vi "TrueRMS.vi"(9 "millisecond multiple":u32, 10 "task/channels in":refnum<k21>) -> (4 "Average":dbl[](graph), 6 "spreadsheet string":string)   [LabVIEW 2021]
uses:
  <vilib>/DAQmx/read.llb/DAQmx Read (Analog 1D Wfm NChan NSamp).vi
  <vilib>/DAQmx/miscellaneous.llb/DAQmx Fill In Error Info.vi
  <vilib>/measure/madcrms.llb/Averaged DC-RMS for N Chan.vi
  <vilib>/measure/madcrms.llb/Basic Averaged DC-RMS for N Chan.vi
  <vilib>/measure/NI_MAPro.lvlib
panel:
  out "Average\n 2":dbl[][](graph)
  out "x*y":dbl[][](array[numeric])
  out "Column 4":i32
  out "Column 3":i32
  out "Column 2":i32
  out "Array":dbl[][](array[numeric])
  out "data":waveform(dbl)[][](array[waveform])
  out "Column":i32
  out "RMS value waveforms":waveform(dbl)[](array[waveform])
  out "DC value waveforms":waveform(dbl)[](array[waveform])
  out "Raw Readings":waveform(dbl)[](graph)
  out "RMS values":dbl[](array[numeric]) format="%.2p"
  out "DC values":dbl[](array[numeric]) format="%.2p"
  out "cycle RMS":dbl[](array[numeric]) format="%.2p"
  out "cycle average":dbl[](array[numeric]) format="%.2p"
  in  "?":bool
  in  "error in":errorcluster
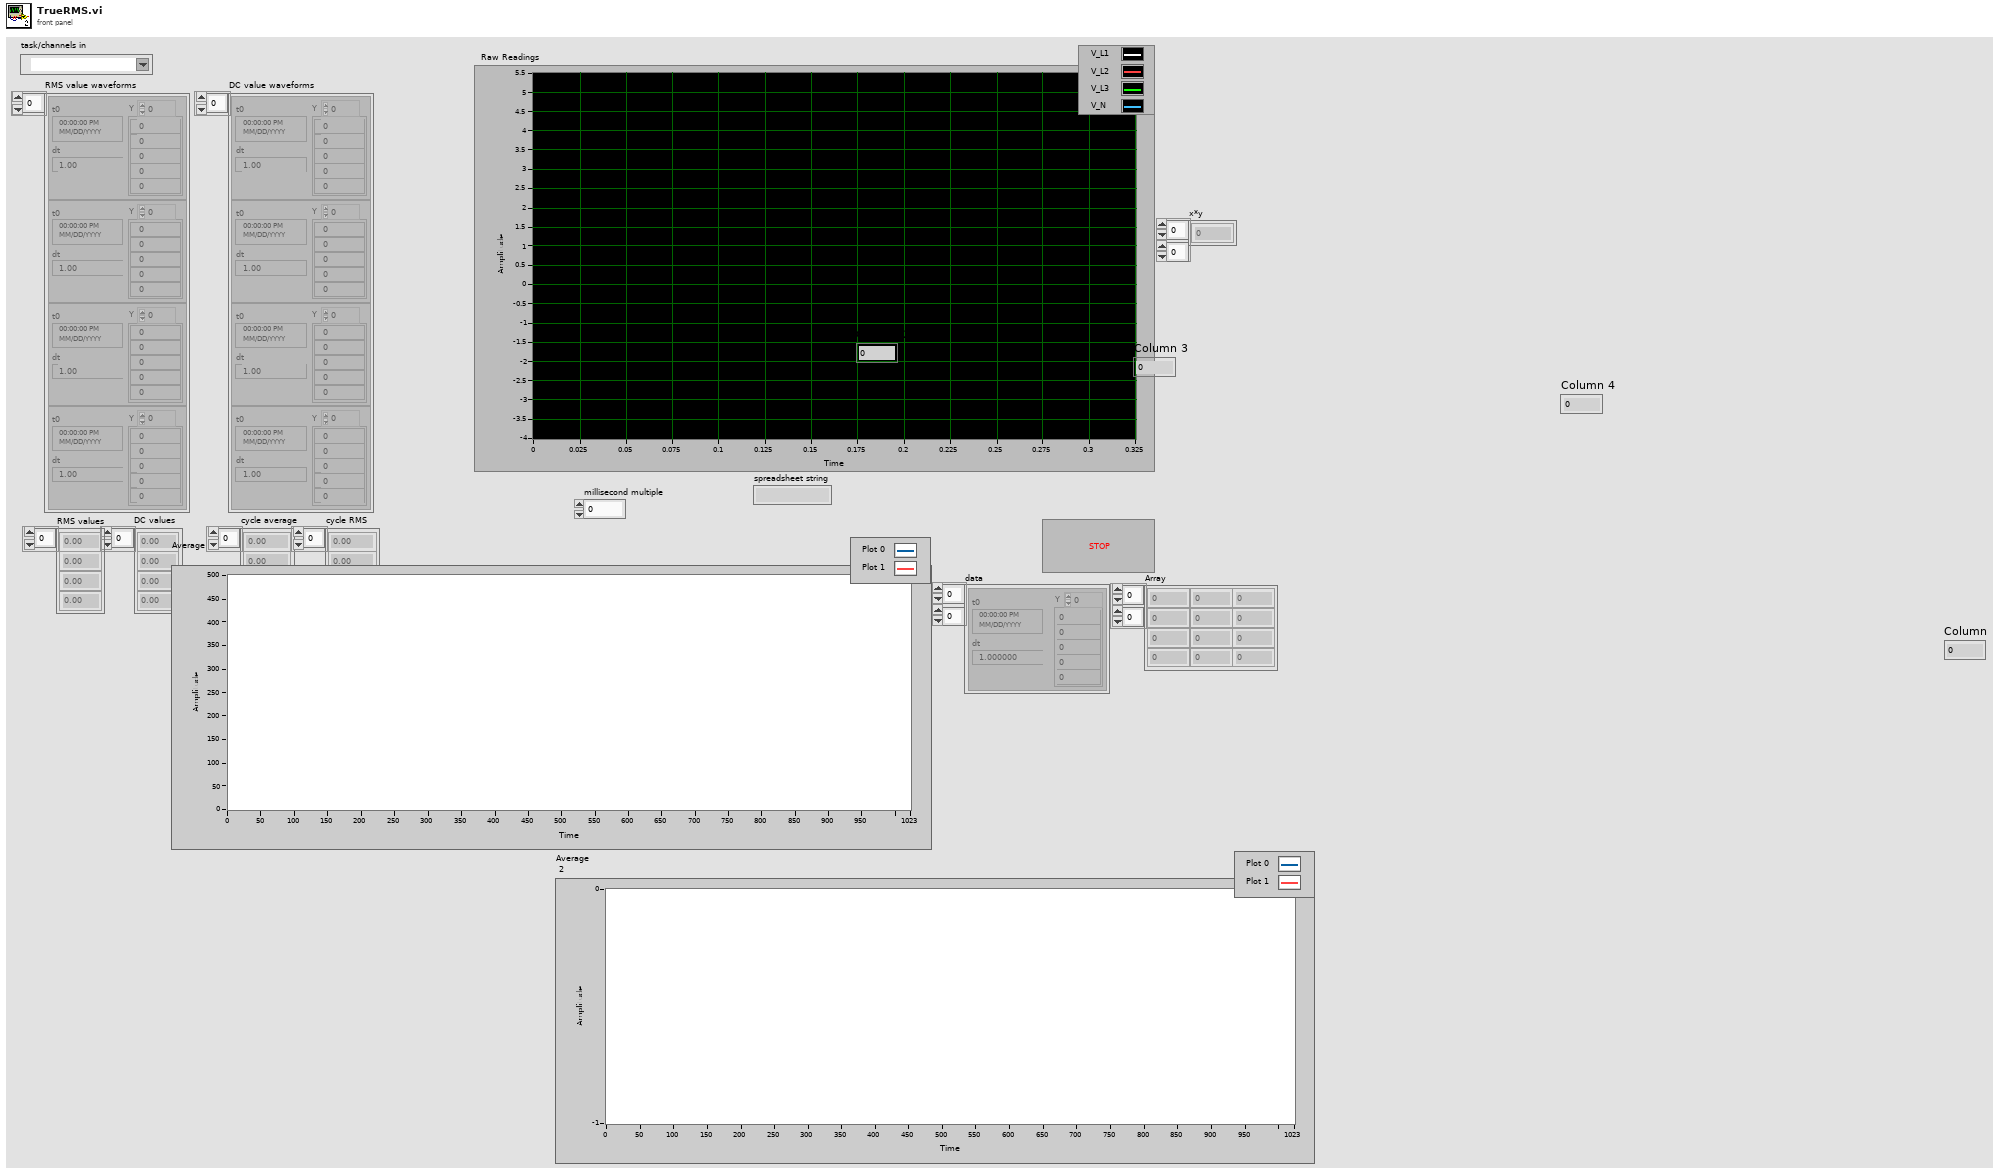
[diagram p1: front panel]
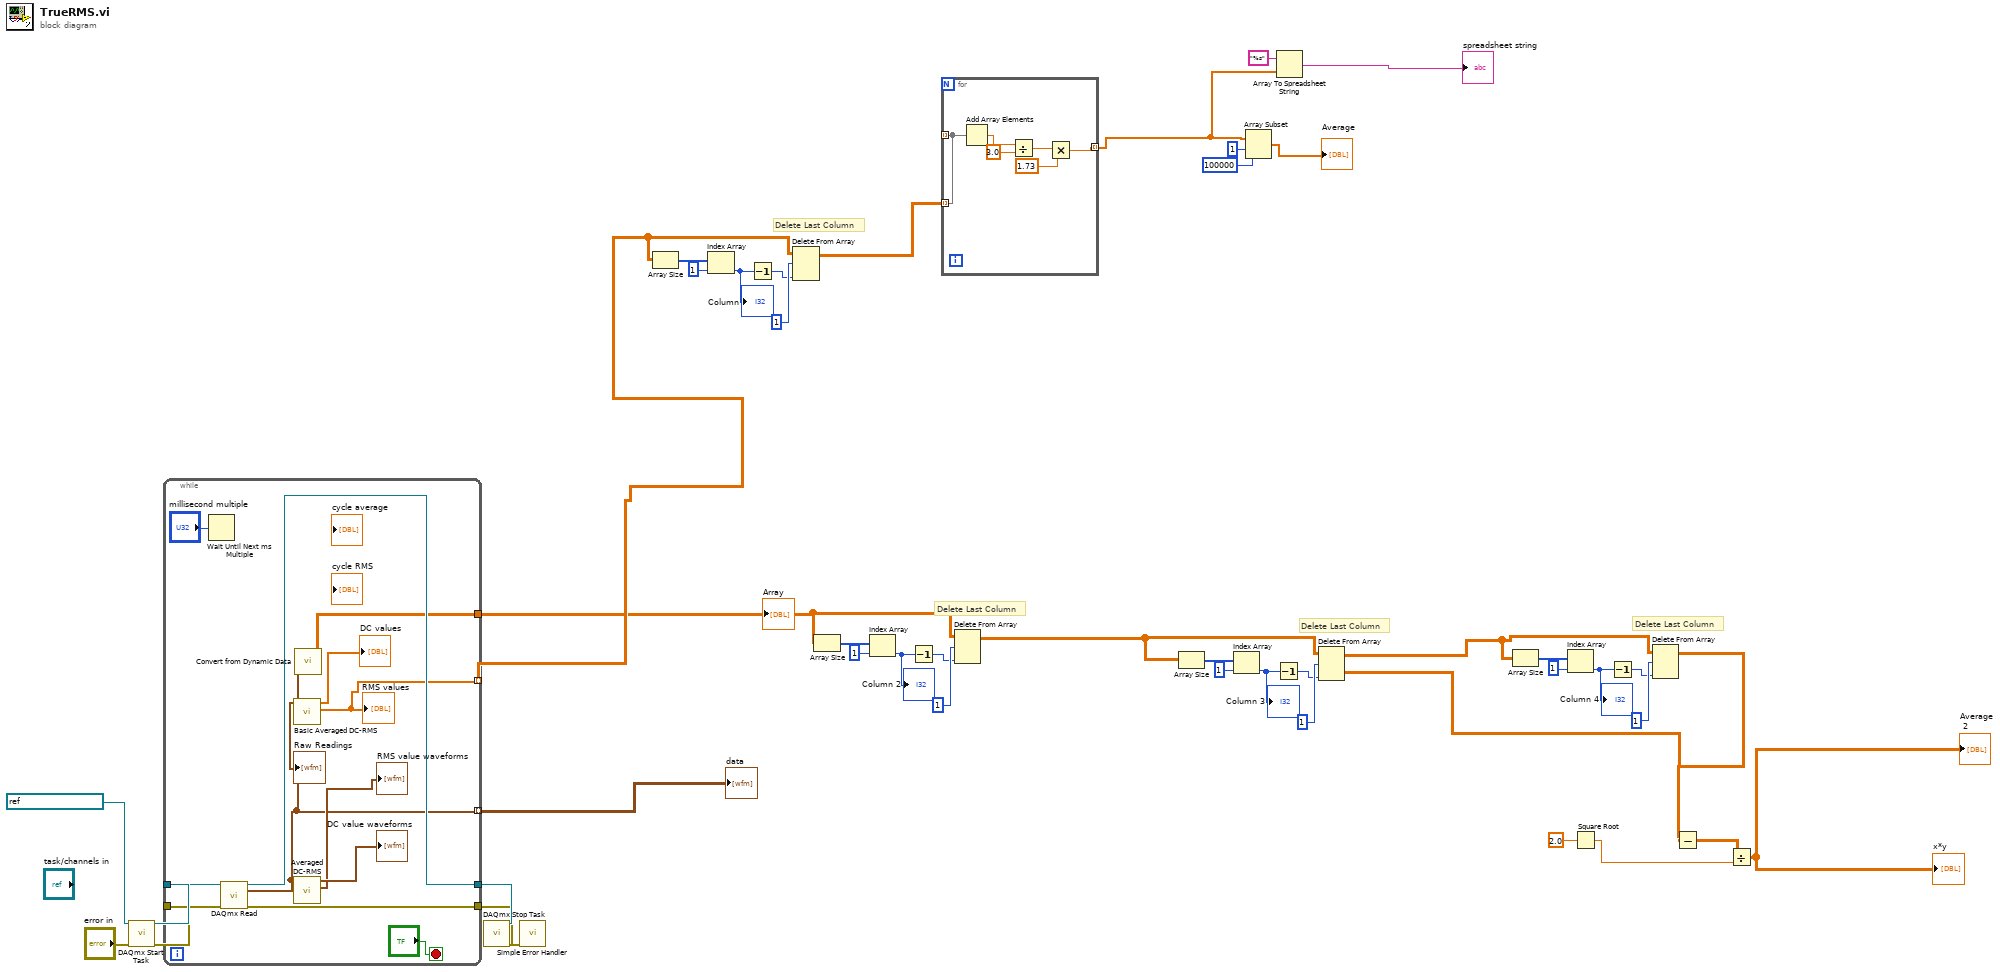
[diagram p0: block diagram]
diagram:
  # "Delete Last Column"
  # "Delete Last Column"
  # "Delete Last Column"
  # "Delete Last Column"
  n1 = call <vilib>:"DAQmx Start Task.vi"("task/channels in"=refnum<k21> "PTS_Cab1k_9244", "error in"="error in") -> ("task out"=w44:refnum<k21>, "error out"=w42:errorcluster)  [unwired: 12 in]
  n2 = while {
    tunnel: w42 -> [w55]
    tunnel: [w54] -> w41
    tunnel: w44 -> [w57]
    tunnel: [w56] -> w43
    tunnel: [w49] -> w29 mode=indexing
    tunnel: [w47] -> w25 mode=indexing
    tunnel: [w46] -> w19
    stop <- "?" stop-if-true
    n3 = Wait Until Next ms Multiple(millisecond multiple="millisecond multiple") -> ()  [unwired: 1 out]
    n4 = call-poly <vilib>:"DAQmx Read.vi"("task/channels in"=w57, "error in"=w55) -> ("task out"=w56:refnum<k21>, "data"=w47:waveform(dbl)[], "error out"=w54:errorcluster)  [unwired: 11 in]
    "Raw Readings" <- w47
    n5 = call-poly <vilib>:"Basic Averaged DC-RMS.vi"("signals in"=w47) -> ("RMS values"=w49:dbl[], "DC values"=→"DC values":dbl[])  [unwired: 7 in, 2 out]
    "RMS values" <- w49
    n6 = call-poly <vilib>:"Averaged DC-RMS.vi"("signals in"=w47) -> ("RMS value waveforms"=→"RMS value waveforms":waveform(dbl)[], "DC value waveforms"=→"DC value waveforms":waveform(dbl)[])  [unwired: 6 in, 3 out]
    n7 = call "Convert from Dynamic Data"("Dynamic Data Type"=w47) -> ("Array"=w46:dbl[][])  [unwired: 3 in]
  }
  "data" <- w25
  "Array" <- w19
  n8 = call <vilib>:"DAQmx Stop Task.vi"("task/channels in"=w43, "error in"=w41) -> ("error out"=w40:errorcluster)  [unwired: 12 in, 1 out]
  n9 = call <vilib>:"Simple Error Handler.vi"("error in (no error)"=w40) -> ()  [unwired: 4 in, 5 out]
  n10 = Array Size(array=w29) -> (size(s)=w38:i32[])
  n11 = Index Array "Index Array"(array=w38, index=1) -> (element=w35:i32)
  "Column" <- w35
  n12 = Decrement(x=w35) -> (x-1=w34:i32)
  n13 = Delete From Array "Delete From Array"(array=w29, length=1 ("index (row)"), index (col)=w34) -> (array with subset deleted=w33:dbl[][])  [unwired: 1 in, 1 out]
  n14 = Array Size(array=w19) -> (size(s)=w24:i32[])
  n15 = Index Array "Index Array"(array=w24, index=1) -> (element=w21:i32)
  "Column 2" <- w21
  n16 = Decrement(x=w21) -> (x-1=w20:i32)
  n17 = for {
    tunnel: [w61] -> _ mode=indexing
    tunnel: [w59] -> w28 mode=indexing
    tunnel: w33 -> [w61] mode=indexing
    n18 = Add Array Elements(numeric array=w61) -> (sum=w63:dbl)
    n19 = Divide(x=w63, y=3.0) -> (x/y=w60:dbl)
    n20 = Multiply(x=w60, y=1.73) -> (x*y=w59:dbl)
  }
  n21 = Delete From Array "Delete From Array"(array=w19, length=1 ("index (row)"), index (col)=w20) -> (array with subset deleted=w13:dbl[][])  [unwired: 1 in, 1 out]
  n22 = Array Size(array=w13) -> (size(s)=w18:i32[])
  n23 = Index Array "Index Array"(array=w18, index=1) -> (element=w15:i32)
  "Column 3" <- w15
  n24 = Array Subset(array=w28, index=1, length=100000) -> (→"Average":dbl[])
  n25 = Decrement(x=w15) -> (x-1=w14:i32)
  n26 = Array To Spreadsheet String(array=w28, 3:"%s" ("format string")) -> (spreadsheet string=→"spreadsheet string":string)  [unwired: 1 in]
  n27 = Delete From Array "Delete From Array"(array=w13, length=1 ("index (row)"), index (col)=w14) -> (deleted portion=w3:dbl[][], array with subset deleted=w7:dbl[][])  [unwired: 1 in]
  n28 = Array Size(array=w7) -> (size(s)=w12:i32[])
  n29 = Index Array "Index Array"(array=w12, index=1) -> (element=w9:i32)
  "Column 4" <- w9
  n30 = Square Root(x=2.0) -> (sqrt(x)=w2:dbl)
  n31 = Decrement(x=w9) -> (x-1=w8:i32)
  n32 = Delete From Array "Delete From Array"(array=w7, length=1 ("index (row)"), index (col)=w8) -> (array with subset deleted=w6:dbl[][])  [unwired: 1 in, 1 out]
  n33 = Subtract(x=w6, y=w3) -> (x-y=w5:dbl[][])
  n34 = Divide(x=w5, y=w2) -> (x/y=→"x*y" →"Average\n 2":dbl[][])
